vi "DSF.Simulation.Custom Device.Get Channel Count.vi"(8 "error in (no error)":errorcluster, 11 "Simulated VeriStand Custom Device in":refnum<class "Simulated VeriStand Custom Device.lvclass">) -> (0 "error out":errorcluster, 2 "Channel Count":u32, 3 "Simulated VeriStand Custom Device out":refnum<class "Simulated VeriStand Custom Device.lvclass">)   [LabVIEW 2016, in "Simulated VeriStand Custom Device.lvclass"]
uses:
  Simulated VeriStand Custom Device.lvclass
  Simulated VeriStand Custom Device.lvclass/Simulated VeriStand Custom Device.ctl
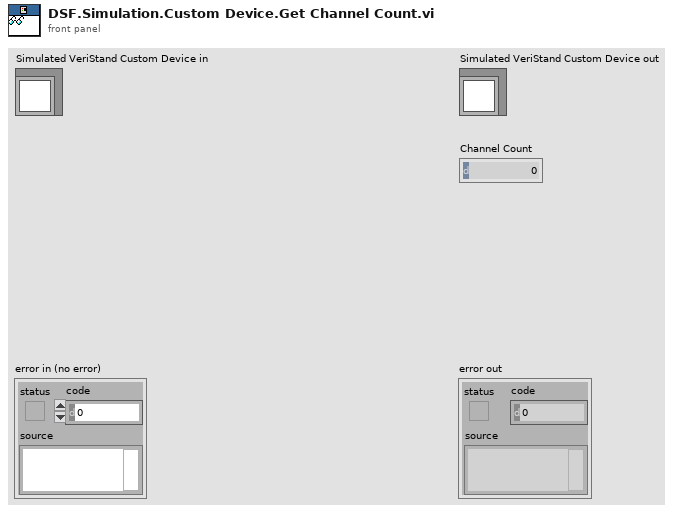
[diagram p1: front panel]
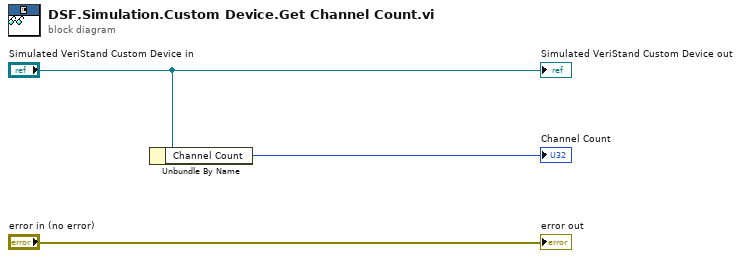
[diagram p0: block diagram]
diagram:
  n1 = Unbundle By Name("Simulated VeriStand Custom Device in") -> ("Channel Count"=→"Channel Count":u32)
  "error out" <- "error in (no error)"
  "Simulated VeriStand Custom Device out" <- "Simulated VeriStand Custom Device in"
